vi "All_Bundled_Resquest1.vi"(5 "Data":string) -> (2 "output_All_Bundled":T2)   [LabVIEW 2021]
uses:
  Controls/Cluster leds 3-5.ctl
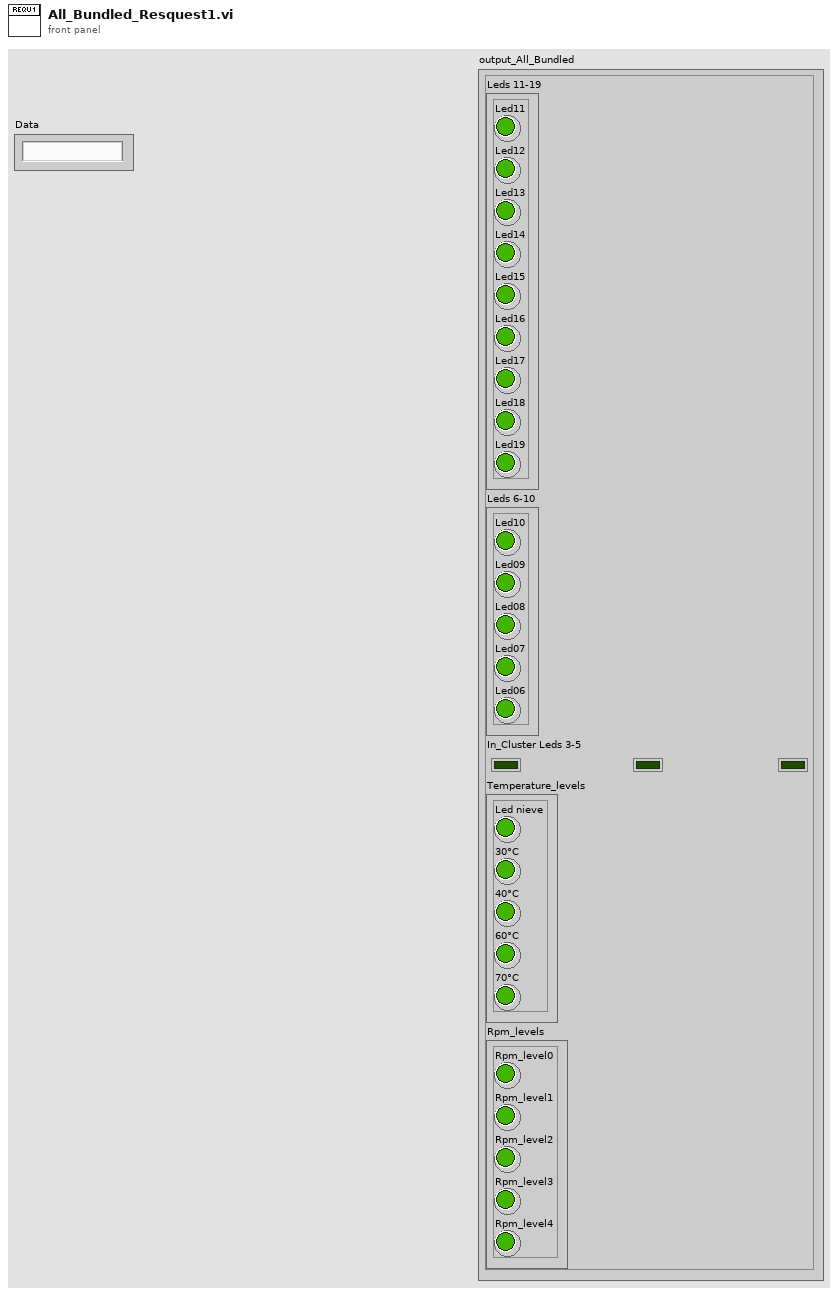
[diagram p1: front panel]
types:
  T1 = typedef "Cluster leds 3-5.ctl" = cluster{"Led03":bool, "Led04":bool, "Led05":bool}
  T2 = cluster{"Leds 11-19":cluster{"Led11":bool, "Led12":bool, "Led13":bool, "Led14":bool, "Led15":bool, "Led16":bool, "Led17":bool, "Led18":bool, "Led19":bool}, "Leds 6-10":cluster{"Led10":bool, "Led09":bool, "Led08":bool, "Led07":bool, "Led06":bool}, "In_Cluster Leds 3-5":T1, "Temperature_levels":cluster{"Led nieve":bool, "30°C":bool, "40°C":bool, "60°C":bool, "70°C":bool}, "Rpm_levels":cluster{"Rpm_level0":bool, "Rpm_level1":bool, "Rpm_level2":bool, "Rpm_level3":bool, "Rpm_level4":bool}}
  T3 = cluster{"Rpm_level0":bool, "Rpm_level1":bool, "Rpm_level2":bool, "Rpm_level3":bool, "Rpm_level4":bool}
  T4 = cluster{"Led nieve":bool, "30°C":bool, "40°C":bool, "60°C":bool, "70°C":bool}
  T5 = cluster{"Led11":bool, "Led12":bool, "Led13":bool, "Led14":bool, "Led15":bool, "Led16":bool, "Led17":bool, "Led18":bool, "Led19":bool}
  T6 = cluster{"Led10":bool, "Led09":bool, "Led08":bool, "Led07":bool, "Led06":bool}
  T7 = cluster{"bit 0":bool, "bit 1":bool, "bit 2":bool, "bit 3":bool, "bit 4":bool, "bit 5":bool, "bit 6":bool, "bit 7":bool}
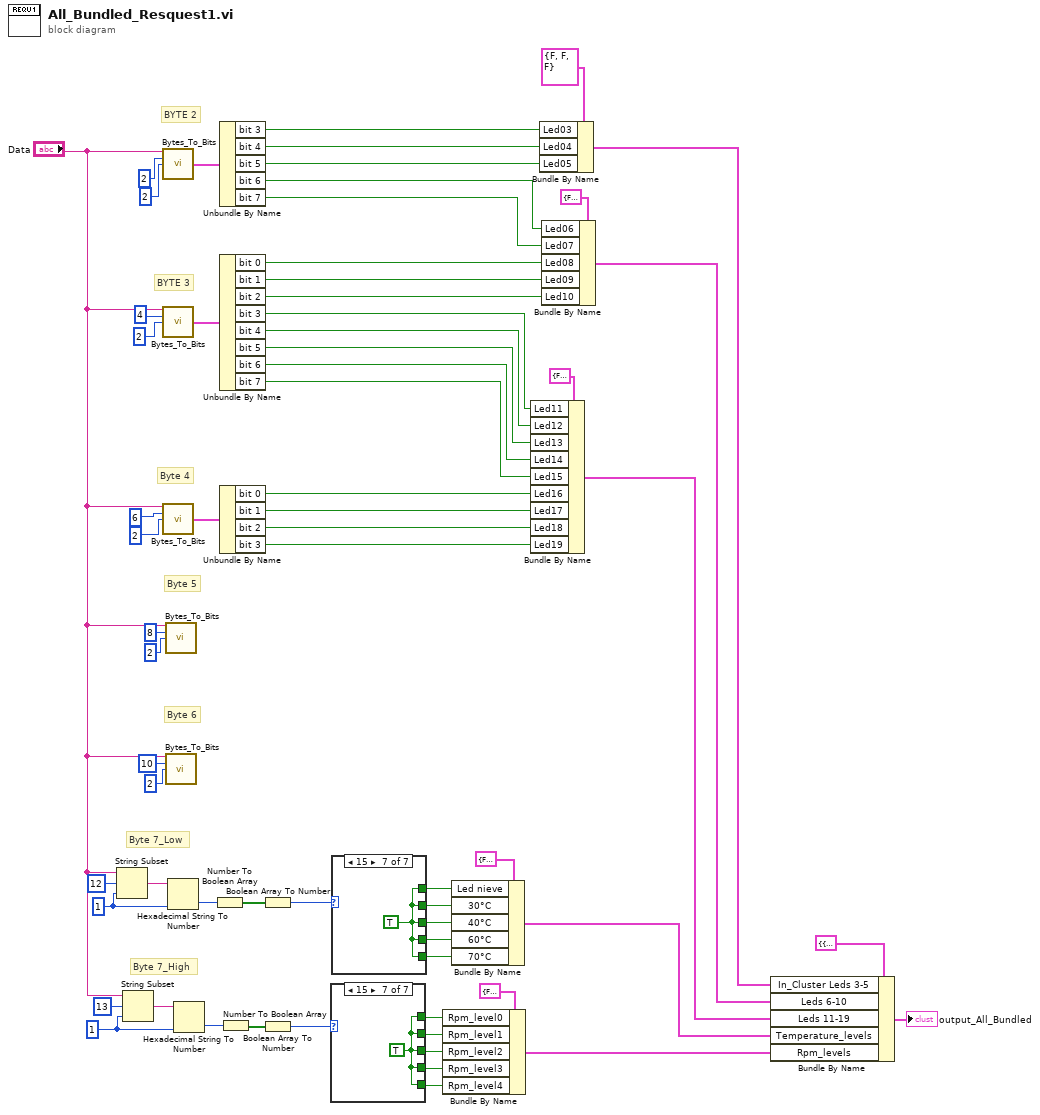
[diagram p0: block diagram]
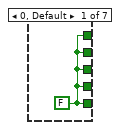
[diagram p2: hidden frame]
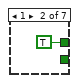
[diagram p3: hidden frame]
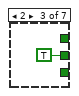
[diagram p4: hidden frame]
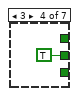
[diagram p5: hidden frame]
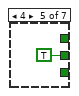
[diagram p6: hidden frame]
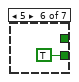
[diagram p7: hidden frame]
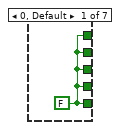
[diagram p8: hidden frame]
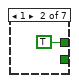
[diagram p9: hidden frame]
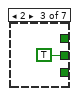
[diagram p10: hidden frame]
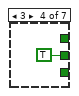
[diagram p11: hidden frame]
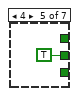
[diagram p12: hidden frame]
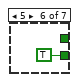
[diagram p13: hidden frame]
diagram:
  w56 = 1 ("length (rest)")
  w61 = 1 ("length (rest)")
  # "Byte 6"
  # "Byte 5"
  # "Byte 4"
  # "BYTE 3"
  # "BYTE 2"
  # "Byte 7_High"
  # "Byte 7_Low"
  n1 = String Subset(string="Data", offset (0)=12, length (rest)=w61) -> (substring=w59:string)
  n2 = String Subset(string="Data", offset (0)=13, length (rest)=w56) -> (substring=w58:string)
  n3 = call "Bytes_To_Bits.vi"("Data"="Data", "offset (0)"=2, "length (rest)"=2) -> ("output cluster"=w29:T7)  [unwired: 12 in]
  n4 = call "Bytes_To_Bits.vi"("Data"="Data", "offset (0)"=4, "length (rest)"=2) -> ("output cluster"=w21:T7)  [unwired: 12 in]
  n5 = call "Bytes_To_Bits.vi"("Data"="Data", "offset (0)"=6, "length (rest)"=2) -> ("output cluster"=w10:T7)  [unwired: 12 in]
  n6 = call "Bytes_To_Bits.vi"("Data"="Data", "offset (0)"=8, "length (rest)"=2) -> ()  [unwired: 12 in, 1 out]
  n7 = call "Bytes_To_Bits.vi"("Data"="Data", "offset (0)"=10, "length (rest)"=2) -> ()  [unwired: 12 in, 1 out]
  n8 = Hexadecimal String To Number(string=w59, default (0uL)=w61) -> (number=w62:i32)  [unwired: 1 in, 1 out]
  n9 = Hexadecimal String To Number(string=w58, default (0uL)=w56) -> (number=w55:i32)  [unwired: 1 in, 1 out]
  n10 = Number To Boolean Array(number=w62) -> (Boolean array=w54:bool[])
  n11 = Unbundle By Name(w29) -> ("bit 3"=w26:bool, "bit 4"=w27:bool, "bit 5"=w28:bool, "bit 6"=w25:bool, "bit 7"=w24:bool)
  n12 = Unbundle By Name(w21) -> ("bit 0"=w18:bool, "bit 1"=w19:bool, "bit 2"=w20:bool, "bit 3"=w17:bool, "bit 4"=w16:bool, "bit 5"=w15:bool, "bit 6"=w14:bool, "bit 7"=w13:bool)
  n13 = Unbundle By Name(w10) -> ("bit 0"=w9:bool, "bit 1"=w8:bool, "bit 2"=w7:bool, "bit 3"=w6:bool)
  n14 = Number To Boolean Array(number=w55) -> (Boolean array=w53:bool[])
  n15 = Boolean Array To Number(Boolean array=w54) -> (number=w52:u32)
  n16 = Boolean Array To Number(Boolean array=w53) -> (number=w46:u32)
  n17 = case shown="15" w46 {
    tunnel: [w66 _ _ _ _ TRUE w72] -> w39
    tunnel: [w66 _ _ _ TRUE _ w72] -> w40
    tunnel: [w66 _ _ TRUE _ _ w72] -> w41
    tunnel: [w66 _ TRUE _ _ _ w72] -> w42
    tunnel: [w66 TRUE _ _ _ _ w72] -> w43
    frame 0, Default {
      w66 = FALSE
    }
    frame 1 {
    }
    frame 2 {
    }
    frame 3 {
    }
    frame 4 {
    }
    frame 5 {
    }
    frame 15 {
      w72 = TRUE
    }
  }
  n18 = case shown="15" w52 {
    tunnel: [w73 _ _ _ _ TRUE w79] -> w51
    tunnel: [w73 _ _ _ TRUE _ w79] -> w50
    tunnel: [w73 _ _ TRUE _ _ w79] -> w49
    tunnel: [w73 _ TRUE _ _ _ w79] -> w48
    tunnel: [w73 TRUE _ _ _ _ w79] -> w47
    frame 0, Default {
      w73 = FALSE
    }
    frame 1 {
    }
    frame 2 {
    }
    frame 3 {
    }
    frame 4 {
    }
    frame 5 {
    }
    frame 15 {
      w79 = TRUE
    }
  }
  n19 = Bundle By Name(cluster=T3 {"Rpm_level0"=FALSE, "Rpm_level1"=FALSE, "Rpm_level2"=FALSE, "Rpm_level3"=FALSE, "Rpm_level4"=FALSE} ("Cluster Rpm_level"), "Rpm_level0"=w43, "Rpm_level1"=w42, "Rpm_level2"=w41, "Rpm_level3"=w40, "Rpm_level4"=w39) -> (w37:T3)
  n20 = Bundle By Name(cluster=T4 {"Led nieve"=FALSE, "30°C"=FALSE, "40°C"=FALSE, "60°C"=FALSE, "70°C"=FALSE} ("Temperature cluster"), "Led nieve"=w47, "30°C"=w48, "40°C"=w49, "60°C"=w50, "70°C"=w51) -> (w36:T4)
  n21 = Bundle By Name(cluster=T5 {"Led11"=FALSE, "Led12"=FALSE, "Led13"=FALSE, "Led14"=FALSE, "Led15"=FALSE, "Led16"=FALSE, "Led17"=FALSE, "Led18"=FALSE, "Led19"=FALSE} ("Cluster Led 11-19"), "Led11"=w17, "Led12"=w16, "Led13"=w15, "Led14"=w14, "Led15"=w13, "Led16"=w9, "Led17"=w8, "Led18"=w7, "Led19"=w6) -> (w35:T5)
  n22 = Bundle By Name(cluster=T1 {"Led03"=FALSE, "Led04"=FALSE, "Led05"=FALSE} ("In_Cluster Leds 3-5"), "Led03"=w26, "Led04"=w27, "Led05"=w28) -> (w33:T1)
  n23 = Bundle By Name(cluster=T6 {"Led10"=FALSE, "Led09"=FALSE, "Led08"=FALSE, "Led07"=FALSE, "Led06"=FALSE} ("Cluster leds 6-10"), "Led06"=w25, "Led07"=w24, "Led08"=w18, "Led09"=w19, "Led10"=w20) -> (w34:T6)
  n24 = Bundle By Name(cluster=T2 {"Leds 11-19"={"Led11"=FALSE, "Led12"=FALSE, "Led13"=FALSE, "Led14"=FALSE, "Led15"=FALSE, "Led16"=FALSE, "Led17"=FALSE, "Led18"=FALSE, "Led19"=FALSE}, "Leds 6-10"={"Led10"=FALSE, "Led09"=FALSE, "Led08"=FALSE, "Led07"=FALSE, "Led06"=FALSE}, "In_Cluster Leds 3-5"={"Led03"=FALSE, "Led04"=FALSE, "Led05"=FALSE}, "Temperature_levels"={"Led nieve"=FALSE, "30°C"=FALSE, "40°C"=FALSE, "60°C"=FALSE, "70°C"=FALSE}, "Rpm_levels"={"Rpm_level0"=FALSE, "Rpm_level1"=FALSE, "Rpm_level2"=FALSE, "Rpm_level3"=FALSE, "Rpm_level4"=FALSE}}, "In_Cluster Leds 3-5"=w33, "Leds 6-10"=w34, "Leds 11-19"=w35, "Temperature_levels"=w36, "Rpm_levels"=w37) -> (→"output_All_Bundled":T2)
